vi "form_monitor.vi"(11 "JSON":string="{\"ch\":0}") -> ()   [LabVIEW 2021]
uses:
  core/host_global_vars.vi
panel:
  in  "Ring":u16(ring) items=["AI 0", "AI 1", "AI 2", "AI 3", "AI 4", "AI 5", "AI 6", "AI 7", "AO 0", "AO 1", "AO 2", "AO 3", "AO 4", "AO 5", "AO 6", "AO 7", "FB 0", "FB 1", "FB 0 error", "FB 1 error"]
  in  "fargs":cluster{"ch":i32}
  out "Waveform Graph":sgl[](graph)
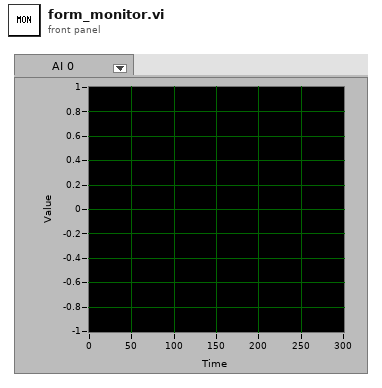
[diagram p1: front panel]
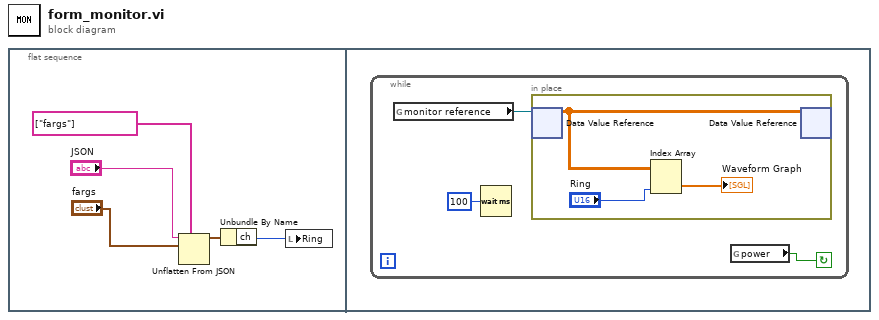
[diagram p0: block diagram]
diagram:
  n1 = flat-sequence {
    frame #0 {
      n2 = Unflatten From JSON(path=string[] ["fargs"], JSON string="JSON", type and defaults="fargs") -> (value=w4:cluster{"ch":i32})  [unwired: 4 in, 1 out]
      n3 = Unbundle By Name(w4) -> ("ch"=w5:i32)
      n4 = local write "Ring"(w5) -> ()
    }
    frame #1 {
      n5 = while {
        stop <- w7 continue-if-true
        n6 = global read "host_global_vars.vi" "monitor reference"() -> (w8:refnum<data-value>)
        n7 = Wait (ms)(milliseconds to wait=u32 100) -> ()  [unwired: 1 out]
        n8 = in-place {
          n9 = in-place-dvr #1(w8) -> (w11:sgl[][])  [unwired: 1 out]
          n10 = Index Array(array=w11, index (col)="Ring") -> (element=→"Waveform Graph":sgl[])  [unwired: 1 in]
          n11 = in-place-dvr #1(w11) -> ()  [unwired: 2 out]
        }
        n12 = global read "host_global_vars.vi" "power"() -> (w7:bool)
      }
    }
  }
